vi "Show Instrument.vi"(8 "error in (no error)":errorcluster, 10 "Test":i32, 11 "Test in":refnum<class "Test.lvclass">) -> (0 "error out":errorcluster, 3 "Test out":refnum<class "Test.lvclass">)   [LabVIEW 2019, in "Test.lvlib" / "Test.lvclass"]
uses:
  Test.lvclass
  Test.lvclass/Test.ctl
  <vilib>/MGI/Panel Manager/Panel Actor/Panel Actor Messages/Show Panel Msg/Show Panel Msg.lvclass
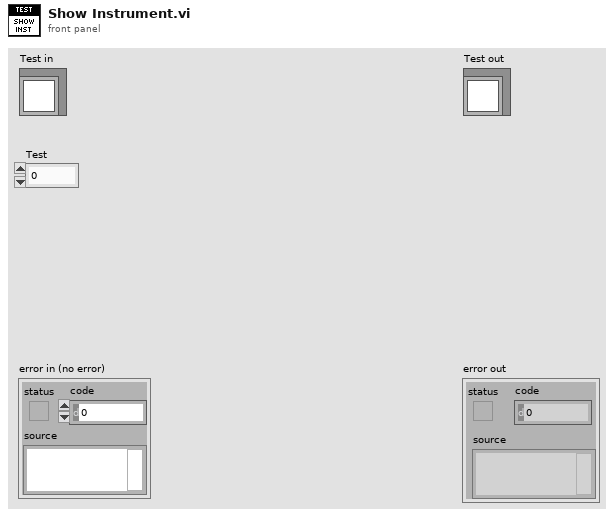
[diagram p1: front panel]
types:
  T1 = map{string, cluster{"Selected Heads":string, "Instrument":refnum<class "Message Enqueuer.lvclass">, "Platform":refnum<class "Message Enqueuer.lvclass">}}
  T2 = cluster{"Selected Heads":string, "Instrument":refnum<class "Message Enqueuer.lvclass">, "Platform":refnum<class "Message Enqueuer.lvclass">}
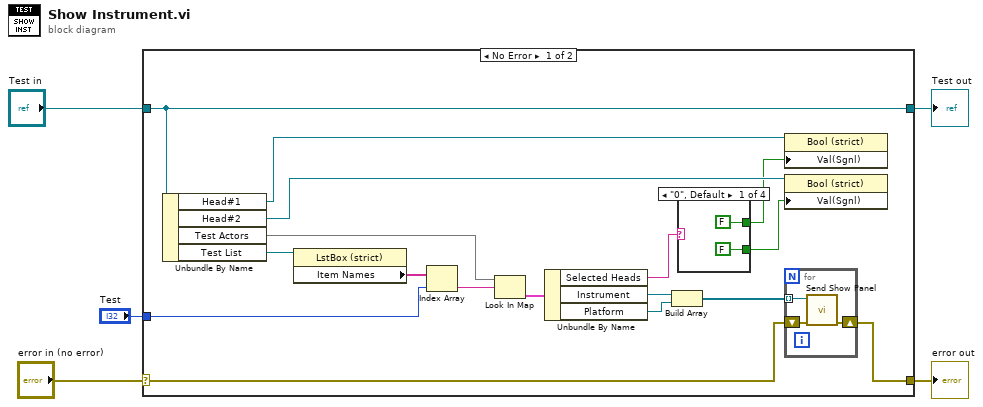
[diagram p0: block diagram]
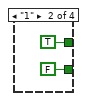
[diagram p2: hidden frame]
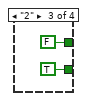
[diagram p3: hidden frame]
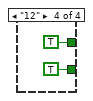
[diagram p4: hidden frame]
diagram:
  n1 = case shown="No Error" "error in (no error)" {
    selector: "error in (no error)" -> [w22 w35]
    tunnel: [w21 w35] -> w4
    tunnel: [w15 w34] -> w3
    tunnel: "Test in" -> [w15 w34]
    tunnel: "Test" -> [w17 _]
    frame No Error {
      n2 = Unbundle By Name(w15) -> ("Head#1"=w12:refnum<vi>, "Head#2"=w13:refnum<vi>, "Test Actors"=w16:T1, "Test List"=w18:refnum<vi>)
      n3 = property class="LstBox (strict)"(reference=w18) -> ("Item Names"=w19:string[])  [unwired: 1 in, 2 out]
      n4 = Index Array(array=w19, index=w17) -> (element=w20:string)
      n5 = Look In Map(map=w16, key=w20) -> (value=w14:T2)  [unwired: 1 in, 1 out]
      n6 = Unbundle By Name(w14) -> ("Selected Heads"=w11:string, "Instrument"=w8:refnum<class "Message Enqueuer.lvclass">, "Platform"=w7:refnum<class "Message Enqueuer.lvclass">)
      n7 = Build Array(w8, w7) -> (w6:refnum<class "Message Enqueuer.lvclass">[])
      n8 = case shown="\"0\", Default" w11 {
        tunnel: [FALSE ("Value") TRUE ("Value") FALSE ("Value") TRUE ("Value")] -> w10
        tunnel: [FALSE ("Value") FALSE ("Value") TRUE ("Value") TRUE ("Value")] -> w9
        frame "0", Default {
        }
        frame "1" {
        }
        frame "2" {
        }
        frame "12" {
        }
      }
      n9 = property class="Bool (strict)"(reference=w12, "Val(Sgnl)"=w10) -> ()  [unwired: 1 in, 2 out]
      n10 = property class="Bool (strict)"(reference=w13, "Val(Sgnl)"=w9) -> ()  [unwired: 1 in, 2 out]
      n11 = for {
        tunnel: w6 -> [w31] mode=indexing
        shift-right: [w32] -> w21
        shift-left: w22 -> [w33]
        n12 = call <vilib>:"Send Show Panel.vi"("Error In"=w33, "Message Enqueuer in"=w31) -> ("Error Out"=w32:errorcluster)  [unwired: 8 in, 1 out]
      }
    }
    frame Error {
    }
  }
  "error out" <- w4
  "Test out" <- w3
